vi "Initialize.vi"(8 "error in (no error)":errorcluster, 11 "GA-Retract-Cmd in":refnum<class "GA-Retract-Cmd.lvclass">) -> (0 "error out":errorcluster, 3 "GA-Retract-Cmd out":refnum<class "GA-Retract-Cmd.lvclass">)   [LabVIEW 2013, in "GA-Retract-Cmd.lvclass"]
uses:
  GA-Retract-Cmd.lvclass
  States/GA-Retracting-State/GrabberArms-RetractingState.lvclass
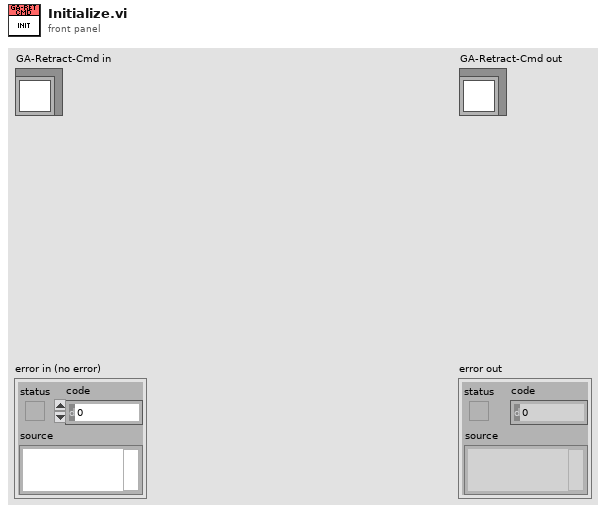
[diagram p1: front panel]
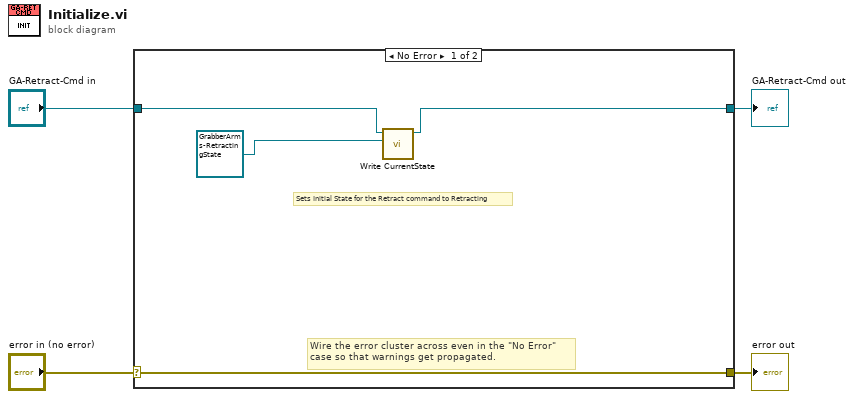
[diagram p0: block diagram]
diagram:
  n1 = case shown="No Error" "error in (no error)" {
    selector: "error in (no error)" -> [w8 w10]
    tunnel: [w8 w10] -> w3
    tunnel: [w6 w9] -> w1
    tunnel: "GA-Retract-Cmd in" -> [w7 w9]
    frame No Error {
      # "Sets Initial State for the Retract command to Retracting"
      # "Wire the error cluster across even in the \"No Error\"\ncase so that warnings get propagated."
      n2 = call-dynamic "Write CurrentState.vi"("State.lvclass"=refnum<class "GrabberArms-RetractingState.lvclass"> refnum ("GrabberArms-RetractingState.lvclass"), "Command in"=w7) -> ("Command out"=w6:refnum<class "GA-Retract-Cmd.lvclass">)  [unwired: 8 in, 1 out]
    }
    frame Error {
    }
  }
  "error out" <- w3
  "GA-Retract-Cmd out" <- w1
